vi "cal_1st_sub_node_x_pos.vi"(0 "Last Function Ref In":refnum<vi>, 5 "Last Function Position":cluster{"Left":i32, "Top":i32}) -> (4 "Last Function Ref Out":refnum<vi>, 10 "1st sub node x position":i32)   [LabVIEW 2018]
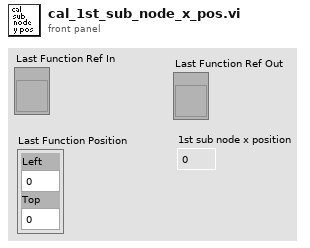
[diagram p1: front panel]
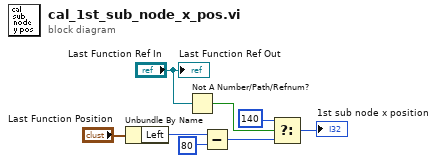
[diagram p0: block diagram]
diagram:
  n1 = Unbundle By Name("Last Function Position") -> ("Left"=w1:i32)
  n2 = Not A Number/Path/Refnum?(number/path/refnum="Last Function Ref In") -> (NaN/Path/Refnum?=w4:bool)
  n3 = Subtract(x=w1, y=80) -> (x-y=w6:i32)
  n4 = Select(t=140, s=w4, f=w6) -> (s? t:f=→"1st sub node x position":i32)
  "Last Function Ref Out" <- "Last Function Ref In"
